vi "Open.vi"(8 "error in (no error)":errorcluster, 11 "PythonSession in":refnum<class "PythonSession.lvclass">) -> (0 "error out":errorcluster, 3 "PythonSession out":refnum<class "PythonSession.lvclass">)   [LabVIEW 2022 SP3, in "PythonWrapper.lvlib" / "PythonSession.lvclass"]
uses:
  PythonSession.lvclass
  _BankAction.ctl
  PythonSession.lvclass/PythonSession.ctl
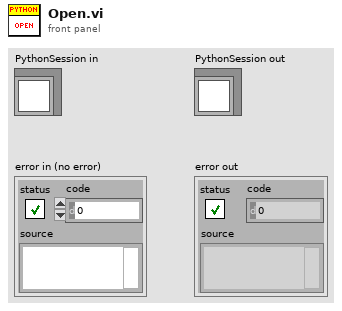
[diagram p1: front panel]
types:
  T1 = typedef "PythonWrapper.lvlib/PythonSession.lvclass/_BankAction.ctl" = enum16{"Add", "Get", "Remove"}
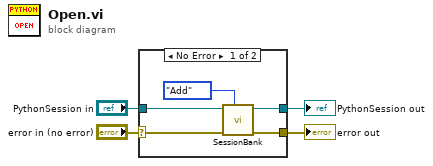
[diagram p0: block diagram]
diagram:
  n1 = case shown="No Error" "error in (no error)" {
    selector: "error in (no error)" -> [w9 w11]
    tunnel: [w8 w11] -> w3
    tunnel: "PythonSession in" -> [w7 w10]
    tunnel: [w6 w10] -> w1
    frame No Error {
      n2 = call "SessionBank.vi"("Action (Get)"=_BankAction."Add" ("Action"), "error in (no error)"=w9, "PythonSession in"=w7) -> ("error out"=w8:errorcluster, "PythonSession out"=w6:refnum<class "PythonSession.lvclass">)  [unwired: 7 in]
    }
    frame Error {
    }
  }
  "error out" <- w3
  "PythonSession out" <- w1
